vi "Find.vi"   [LabVIEW 2014, in "nisyscfg.lvlib"]
doc: "Finds systems and their installed hardware."
uses:
  nisyscfg.lvlib
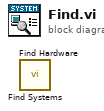
[diagram p0: block diagram]
diagram:
  n1 = call "Find Systems.vi"() -> ()  [unwired: 9 in, 3 out]
  n2 = call "Find Hardware.vi"() -> ()  [unwired: 8 in, 4 out]
